vi "4 channels no handoff DAQAsst.vi"() -> ()   [LabVIEW 2025]
panel:
  out "error out 2":errorcluster
  out "error out":errorcluster
  out "Blue":bool
  in  "Loop Time (ms)":u32=50
  in  "U":bool
  out "Yellow":bool
  out "Orange":bool
  out "Pink":bool
  in  "stop":bool
  # "TO RIGHT"
  # "TO LEFT"
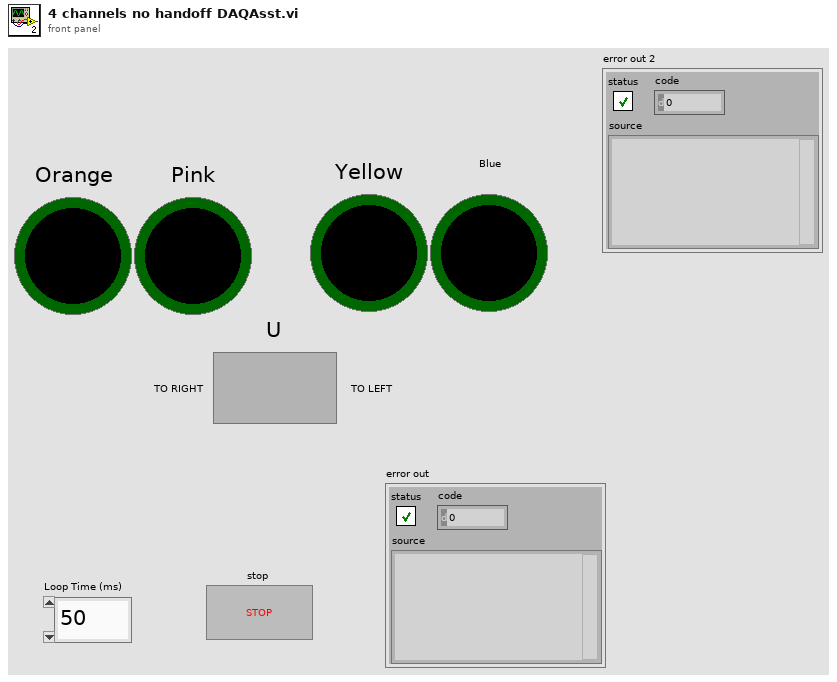
[diagram p1: front panel]
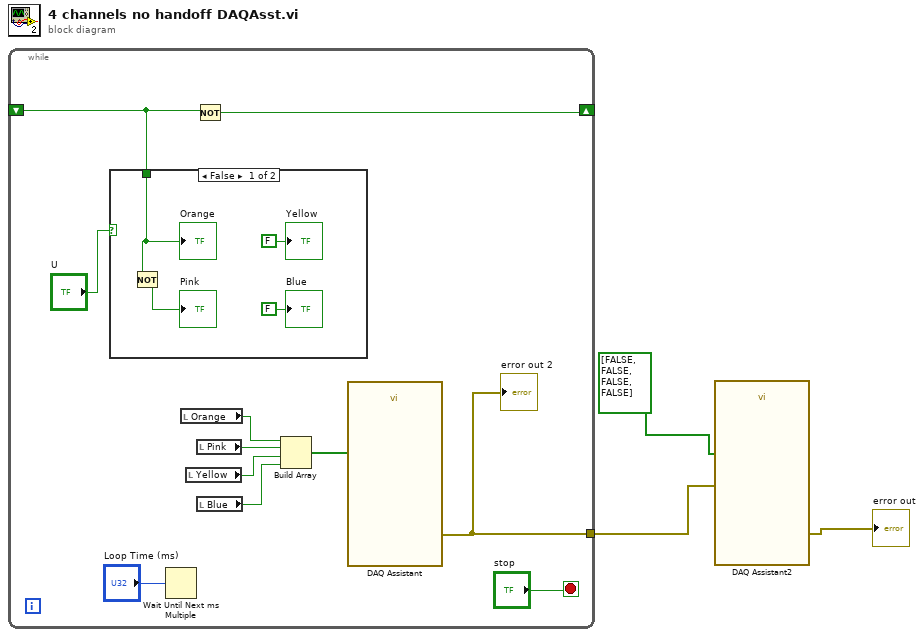
[diagram p0: block diagram]
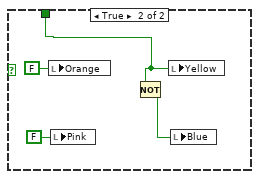
[diagram p2: hidden frame]
diagram:
  n1 = while {
    shift-right: [w13] -> _
    shift-left: _ -> [w11]
    tunnel: [w4] -> w3
    stop <- "stop" stop-if-true
    n2 = case shown="False" "U" {
      tunnel: w11 -> [w16 w22]
      frame False {
        n3 = Not(x=w16) -> (.not. x?=→"Pink":bool)
        "Orange" <- w16
        "Yellow" <- FALSE ("Yellow")
        "Blue" <- FALSE ("Blue")
      }
      frame True {
        n4 = local write "Orange"(FALSE ("Orange")) -> ()
        n5 = local write "Pink"(FALSE ("Pink")) -> ()
        n6 = Not(x=w22) -> (.not. x?=w19:bool)
        n7 = local write "Yellow"(w22) -> ()
        n8 = local write "Blue"(w19) -> ()
      }
    }
    n9 = Wait Until Next ms Multiple(millisecond multiple="Loop Time (ms)") -> ()  [unwired: 1 out]
    n10 = local read "Orange"() -> (w10:bool)
    n11 = local read "Yellow"() -> (w8:bool)
    n12 = Not(x=w11) -> (.not. x?=w13:bool)
    n13 = local read "Pink"() -> (w9:bool)
    n14 = local read "Blue"() -> (w7:bool)
    n15 = Build Array(w10, w9, w8, w7) -> (w5:bool[])
    n16 = call "DAQ Assistant"("data"=w5) -> ("error out"=w4:errorcluster)  [unwired: 17 in, 1 out]
    "error out 2" <- w4
  }
  n17 = call "DAQ Assistant2"("data"=bool[] [FALSE, FALSE, FALSE, FALSE], "error in"=w3) -> ("error out"=→"error out":errorcluster)  [unwired: 16 in, 1 out]
